vi "encoders.vi"() -> (0 "Lift":cluster{"Distance":dbl, "Rate":dbl}, 1 "Front Right Wheel":cluster{"Distance":dbl, "Rate":dbl}, 2 "Front Left Wheel":cluster{"Distance":dbl, "Rate":dbl}, 3 "Back Left Wheel":cluster{"Distance":dbl, "Rate":dbl}, 4 "Container Arm":cluster{"Distance":dbl, "Rate":dbl}, 5 "Back Right Wheel":cluster{"Distance":dbl, "Rate":dbl}, 7 "Center Wheel":cluster{"Distance":dbl, "Rate":dbl})   [LabVIEW 2015]
uses:
  <vilib>/Rock Robotics/Network Tables/NT Read Numeric Array.vi
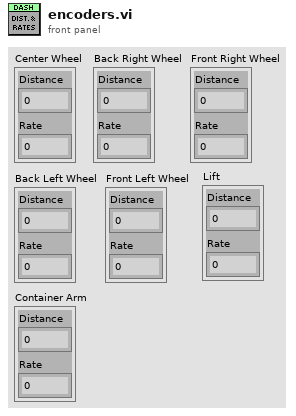
[diagram p1: front panel]
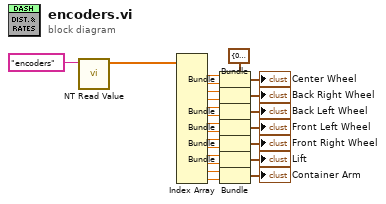
[diagram p0: block diagram]
diagram:
  w8 = cluster{"Distance":dbl, "Rate":dbl} {"Distance"=0.0, "Rate"=0.0}
  n1 = call-poly <vilib>:"NT Read Value.vi"("Name"="encoders") -> ("Numeric Array"=w23:dbl[])  [unwired: 9 in, 1 out]
  n2 = Index Array(array=w23) -> (element #1=w21:dbl, element #2=w22:dbl, element #3=w20:dbl, element #4=w19:dbl, element #5=w18:dbl, element #6=w17:dbl, element #7=w16:dbl, element #8=w15:dbl, element #9=w14:dbl, element #10=w13:dbl, element #11=w12:dbl, element #12=w10:dbl, element #13=w11:dbl, element #14=w9:dbl)  [unwired: 14 in]
  n3 = Bundle(cluster=w8, "Distance"=w21, "Rate"=w22) -> (→"Center Wheel":cluster{"Distance":dbl, "Rate":dbl})
  n4 = Bundle(cluster=w8, "Distance"=w20, "Rate"=w19) -> (→"Back Right Wheel":cluster{"Distance":dbl, "Rate":dbl})
  n5 = Bundle(cluster=w8, "Distance"=w18, "Rate"=w17) -> (→"Back Left Wheel":cluster{"Distance":dbl, "Rate":dbl})
  n6 = Bundle(cluster=w8, "Distance"=w16, "Rate"=w15) -> (→"Front Left Wheel":cluster{"Distance":dbl, "Rate":dbl})
  n7 = Bundle(cluster=w8, "Distance"=w14, "Rate"=w13) -> (→"Front Right Wheel":cluster{"Distance":dbl, "Rate":dbl})
  n8 = Bundle(cluster=w8, "Distance"=w12, "Rate"=w10) -> (→"Lift":cluster{"Distance":dbl, "Rate":dbl})
  n9 = Bundle(cluster=w8, "Distance"=w11, "Rate"=w9) -> (→"Container Arm":cluster{"Distance":dbl, "Rate":dbl})
